vi "Grant Motor Control.vi"() -> ()   [LabVIEW 2012]
doc: "Compressor with Cylinder \n\nThis example shows how to control a compressor, extend and retract a cylinder, and optionally use a limit switch to retract automatically.\n\nThis example works with the NI 9403 module connected to a Digital Sidecar. The Digital Sidecar should have 12V applied to the WAGO connector. A SPIKE relay is used to turn the compressor on and off. The PWM type input on the SPIKE should be wired to RELAY 1 on the Digital Sidecar. The GND and 12V inputs on the SPIKE should get power from the battery through a 20A fuse on the Power Distribution Board. The M+ and M- outputs from the SPIKE should be wired to the compressor. Wire M+ to the red compressor wire, and M- to the black compressor wire. The Pressure Switch is wired to DIGITAL I/O 1. This input determines when the SPIKE relay gets energized to run the compressor. The Limit Switch is wired to DIGITAL I/O 2. It causes the cylinder to retract when the Auto Retract button is pressed.\n\nThis example also uses the Solenoid Breakout connected to the NI 9472 to control the SMC double solenoid valve. From the Solenoid Breakout, channel 1 is wired to terminal A on the valve, and channel 2 is wired to terminal B on the valve.\n\nRefer to the Pneumatics Manual for air connections. Your pneumatics setup should include a compressor, pressure switch, tank, regulator, valve, flow controls, cylinder, plug valve, etc.\n\nTo run this example you should have a pneumatic system with air pressure connected to the P input on the SMC double solenoid valve. The A output of the valve should be connected via a flow control to the backend of a cylinder. The B output of the valve should be connected via a flow control to the frontend of a cylinder. When the cylinder is extended, it should physically depress the Limit Switch.\n\nWith the VI running, pressing the Extend button will push the cylinder shaft out, and pressing the Retract button will pull it back. Notice that the Extend and Retract buttons have their Mechanical Action set to Latch When Pressed. This means they stay pressed (ON) until they are read by the program, then they return to the OFF position. This works because once the SMC solenoid valve is pulled one direction, it stays in that position until it is pulled in the opposite direction - it only needs to be momentarily energized. The Auto Retract button can be used to make the cylinder return automatically. With the Auto Retract button ON, pressing the Extend button will push the cylinder out, and it will retract when it hits the limit switch."
uses:
  <vilib>/Rock Robotics/WPI/MotorControl/WPI_MotorControlOpen Talon.vi
  <vilib>/Rock Robotics/SystemInterfaces/DIO/FPGA_DIOPWMChannel.ctl
panel:
  in  "Run Time":u32
  in  "On/Off 2":bool
  in  "Left Joystick 2":dbl(slide) min=-1.0 max=1.0 step=0.1 scale=-1.0..1.0
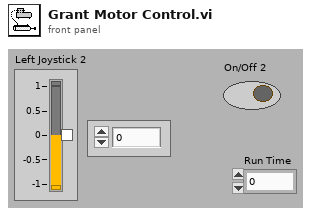
[diagram p1: front panel]
types:
  T1 = typedef "FPGA_DIOPWMChannel.ctl" = enum8{"PWM 1", "PWM 2", "PWM 3", "PWM 4", "PWM 5", "PWM 6", "PWM 7", "PWM 8", "PWM 9", "PWM 10", "Invalid"}
  T2 = typedef "WPI_MotorControlDeviceRef.ctl" = cluster{"DeviceStatus":errorcluster, "Type":enum16{"PWM", "CAN"}, "PWM":cluster{"Digital Module":T3, "PWM Channel":T1, "DeadBand":T4}, "CAN":cluster{"Device Number":u8, "Control Mode":T5, "Semaphore":T6, "Max Vout":dbl}, "Invert":bool, "TransformRef":T7, "InvTransformRef":T7}
  T3 = typedef "FPGA_TypedefDigitalModule.ctl" = enum16{"Digital Module 1", "Digital Module 2"}
  T4 = typedef "WPI_PWMDeadband.ctl" = cluster{"Name":string, "maxPositivePwm":i32, "minPositivePwm":i32, "centerPwm":i32, "maxNegativePwm":i32, "minNegativePwm":i32, "angularRange":u16}
  T5 = typedef "WPI_CANJaguar_ControlMode.ctl" = enum8{"Percent VBus", "Current", "Speed", "Position", "Voltage"}
  T6 = typedef "Semaphore RefNum" = refnum<k1>
  T7 = typedef "WPI_PWMTransform_ConPane.ctl" = refnum<vi>
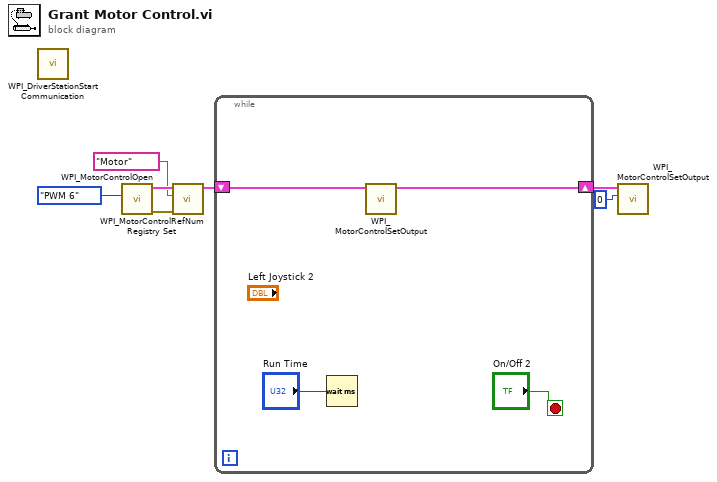
[diagram p0: block diagram]
diagram:
  n1 = call <vilib>:"WPI_DriverStationStart Communication.vi"() -> ()  [unwired: 12 in]
  n2 = call-poly <vilib>:"WPI_MotorControlOpen.vi"("PWM Channel"=FPGA_DIOPWMChannel."PWM 6") -> ("error out"=w6:errorcluster, "MotorControlDeviceRef"=w5:T2)  [unwired: 9 in]
  n3 = call <vilib>:"WPI_MotorControlRefNum Registry Set.vi"("error in (no error)"=w6, "refnum name"="Motor", "MotorControlDevRef"=w5) -> ("MotorControlDevRef"=w4:T2)  [unwired: 7 in, 1 out]
  n4 = while {
    shift-right: [w10] -> w1
    shift-left: w4 -> [w11]
    stop <- "On/Off 2" stop-if-true
    n5 = Wait (ms)(milliseconds to wait="Run Time") -> ()  [unwired: 1 out]
    n6 = call <vilib>:"WPI_MotorControlSetOutput.vi"("MotorControlDevRef"=w11) -> ("MotorControlDevRef"=w10:T2)  [unwired: 8 in, 2 out]
  }
  n7 = call <vilib>:"WPI_MotorControlSetOutput.vi"("Output"=0, "MotorControlDevRef"=w1) -> ()  [unwired: 7 in, 3 out]
